vi "Close.vi"(8 "error in (no error)":errorcluster, 11 "Tektronix DMM4020 in":refnum<class "Tektronix DMM4020.lvclass">) -> (0 "error out":errorcluster, 3 "Tektronix DMM4020 out":refnum<class "Tektronix DMM4020.lvclass">)   [LabVIEW 2014, in "Generic Power Analyzer.lvlib" / "Tektronix DMM4020.lvlib" / "Tektronix DMM4020.lvclass"]
uses:
  Tektronix DMM4020.lvclass
  Generic Power Analyzer/Generic Power Analyzer.lvclass
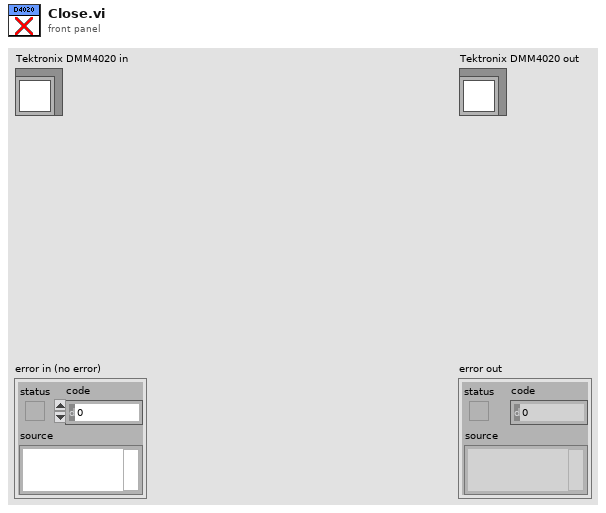
[diagram p1: front panel]
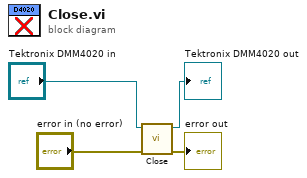
[diagram p0: block diagram]
diagram:
  n1 = call-parent "Close.vi"("error in (no error)"="error in (no error)", "Generic Power Analyzer in"="Tektronix DMM4020 in") -> ("error out"=→"error out":errorcluster, "Generic Power Analyzer out"=→"Tektronix DMM4020 out":refnum<class "Tektronix DMM4020.lvclass">)  [unwired: 8 in]
